vi "Example Cluster.vi"() -> ()   [LabVIEW 2015]
panel:
  out "Employee Record Out":T1={"First Name"="Jennifer", "Preferred Name"="Mc", "Surname"="Swift", "Department"=enum."Finance", "Employment Status"=enum."Part Time", "Start Date"=timestamp(3565024425.501588 s since 1904-01-01), "Normal Working Location"=enum."Working From Home"} {"Start Date" format="%<%x %.3X>T"}
  out "Years in Service":dbl=4.027401130969894
  out "Full Name":string="Jennifer (Jenny) Swift"
  in  "Employee Record In":T1={"First Name"="Jennifer", "Preferred Name"="Jenny", "Surname"="Swift", "Department"=enum."Finance", "Employment Status"=enum."Part Time", "Start Date"=timestamp(3565024425.501588 s since 1904-01-01), "Normal Working Location"=enum."Working in Office"} {"Start Date" format="%<%x %.3X>T"}
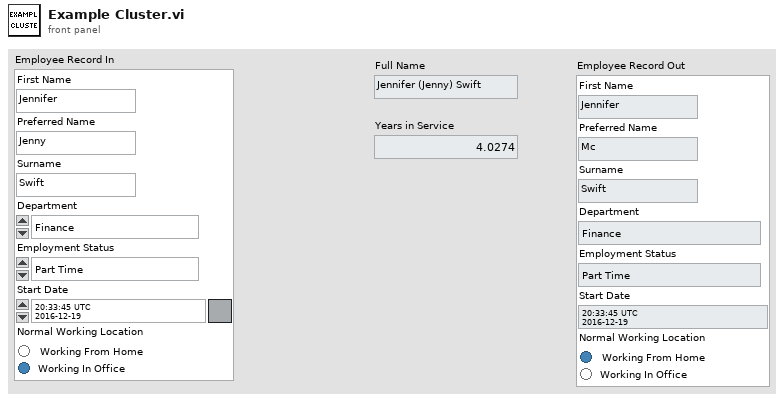
[diagram p1: front panel]
types:
  T1 = cluster{"First Name":string, "Preferred Name":string, "Surname":string, "Department":enum16{"Research and Development", "Technical Support", "Sales", "Management", "Finance", "Other"}, "Employment Status":enum16{"Full Time", "Part Time", "No Longer Employed", "Probation", "Other"}, "Start Date":timestamp, "Normal Working Location":enum32{"Working From Home", "Working in Office"}}
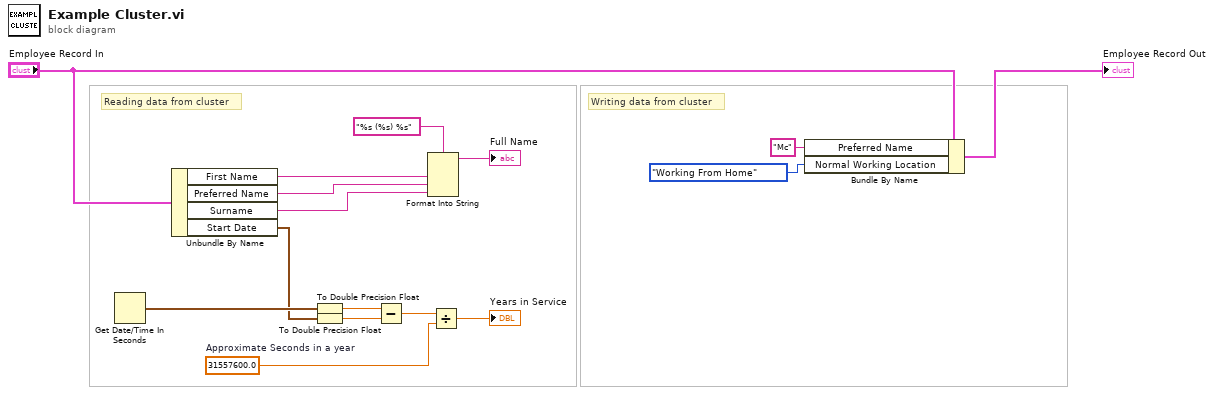
[diagram p0: block diagram]
diagram:
  w14 = 31557600.0  # Approximate Seconds in a year
  # "Writing data from cluster"
  # "Reading data from cluster"
  n1 = Get Date/Time In Seconds() -> (seconds since 1Jan1904=w16:timestamp)
  n2 = Unbundle By Name "Unbundle By Name"("Employee Record In") -> ("First Name"=w8:string, "Preferred Name"=w7:string, "Surname"=w6:string, "Start Date"=w12:timestamp)
  n3 = To Double Precision Float(number=w16) -> (double precision float=w10:dbl)
  n4 = To Double Precision Float(number=w12) -> (double precision float=w11:dbl)
  n5 = Subtract(x=w10, y=w11) -> (x-y=w15:dbl)
  n6 = Format Into String(format string="%s (%s) %s", w8, w7, w6) -> (resulting string=→"Full Name":string)  [unwired: 2 in, 1 out]
  n7 = Divide(x=w15, y=w14) -> (x/y=→"Years in Service":dbl)
  n8 = Bundle By Name "Bundle By Name"(cluster="Employee Record In", "Preferred Name"="Mc", "Normal Working Location"=enum32{"Working From Home", "Working in Office"}."Working From Home") -> (→"Employee Record Out":T1)
